vi "GT 2D Compare Pulse.vi"(6 "time":i16, 7 "outputType":i16, 8 "error in (no error)":errorcluster caption="错误输入（无错误）", 9 "level":i16, 10 "chn":i16, 11 "cardNum":i16) -> (0 "error out":errorcluster caption="错误输出", 3 "function return":i16)   [LabVIEW 2020, in "gts.lvlib"]
doc: "GT_API GT_2DComparePulse(short cardNum,short chn,short level,short outputType,short time);"
uses:
  gts.lvlib
  dll/32bit/multi_card/gts.dll
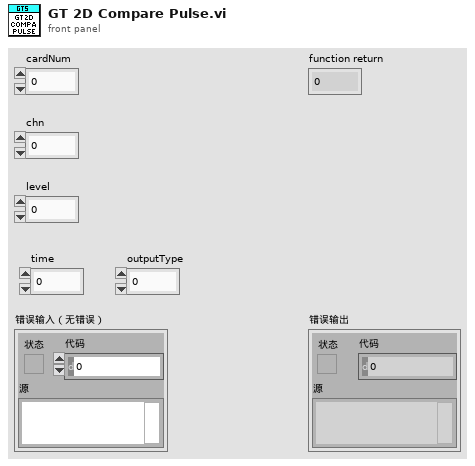
[diagram p1: front panel]
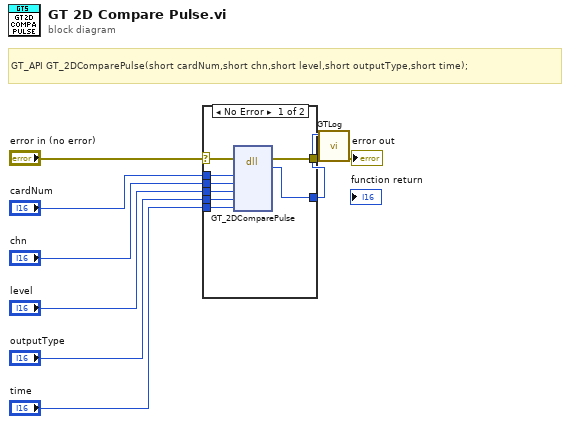
[diagram p0: block diagram]
diagram:
  # "GT_API GT_2DComparePulse(short cardNum,short chn,short level,short outputType,short time);"
  n1 = case shown="No Error" "error in (no error)" {
    selector: "error in (no error)" -> [w11 w18]
    tunnel: [w17 _] -> w1
    tunnel: "cardNum" -> [w16 _]
    tunnel: "chn" -> [w15 _]
    tunnel: "level" -> [w14 _]
    tunnel: "outputType" -> [w13 _]
    tunnel: "time" -> [w12 _]
    tunnel: [w10 w18] -> w3
    frame No Error {
      n2 = dll-call lib="C:/1228/dll/32bit/multi_card/gts.*" fn="GT_2DComparePulse"(error in=w11, "cardNum"=w16, "chn"=w15, "level"=w14, "outputType"=w13, "time"=w12) -> (error out=w10:errorcluster, w17:i16)  [unwired: 7 in, 1 out]
    }
    frame Error {
    }
  }
  n3 = call "GTLog.vi"("error in (no error)"=w3, "Numeric"=w1) -> ("error out"=→"error out":errorcluster)  [unwired: 9 in]
